vi "isRefValid.vi"(8 "error in (no error)":errorcluster, 11 "xwpfDocument in":refnum<class "xwpfDocument.lvclass">) -> (0 "error out":errorcluster, 3 "xwpfDocument out":refnum<class "xwpfDocument.lvclass">)   [LabVIEW 2017, in "Word_Specific.lvlib" / "xwpfDocument.lvclass"]
uses:
  xwpfDocument.lvclass
  xwpfDocument.lvclass/xwpfDocument.ctl
  <vilib>/Utility/error.llb/Error Cluster From Error Code.vi
  <vilib>/ErrorRing/Error Ring.xnode
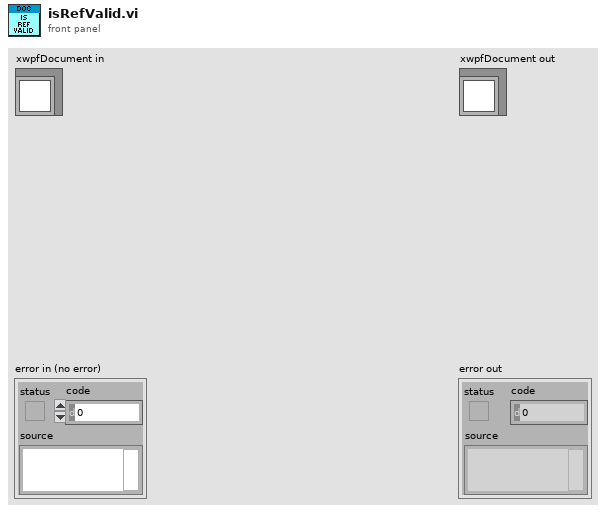
[diagram p1: front panel]
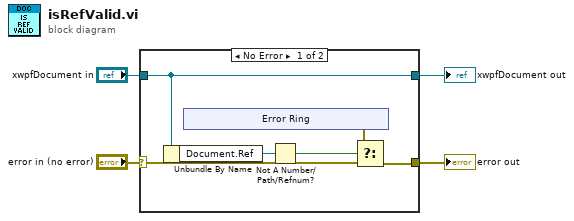
[diagram p0: block diagram]
diagram:
  n1 = case shown="No Error" "error in (no error)" {
    selector: "error in (no error)" -> [w7 w17]
    tunnel: [w6 w17] -> w2
    tunnel: [w10 w16] -> w1
    tunnel: "xwpfDocument in" -> [w10 w16]
    frame No Error {
      n2 = Unbundle By Name(w10) -> ("Document.Ref"=w5:refnum<k24>)
      n3 = xnode "Error Ring"() -> ("error out"=w8:errorcluster)
      n4 = Not A Number/Path/Refnum?(number/path/refnum=w5) -> (NaN/Path/Refnum?=w9:bool)
      n5 = Select(t=w8, s=w9, f=w7) -> (s? t:f=w6:errorcluster)
    }
    frame Error {
    }
  }
  "error out" <- w2
  "xwpfDocument out" <- w1
